vi "Ctor.vi"(8 "error in (no error)":errorcluster) -> (0 "error out":errorcluster, 3 "PlatformManager out":refnum<class "PlatformManager.lvclass">)   [LabVIEW 2020, in "PicoG-Core.lvlib" / "PlatformManager.lvclass"]
uses:
  PlatformManager.lvclass
  Ref Data.ctl
  Platform/Platform.lvclass
  PlatformManager.lvclass/PlatformManager.ctl
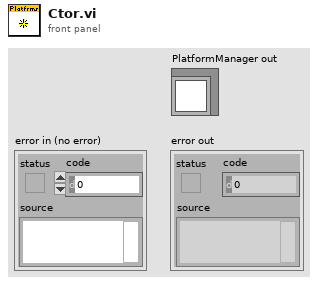
[diagram p1: front panel]
types:
  T1 = typedef "PicoG-Core.lvlib/PlatformManager.lvclass/Ref Data.ctl" = cluster{"Platforms":refnum<class "Platform.lvclass">[]}
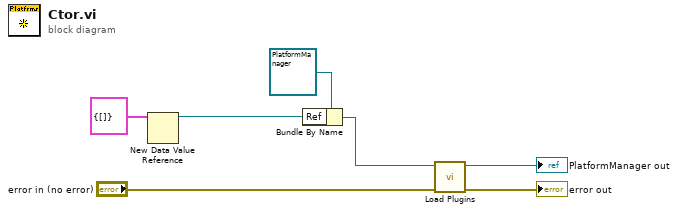
[diagram p0: block diagram]
diagram:
  n1 = New Data Value Reference(data value=T1 {"Platforms"=[]} ("Ref Data")) -> (data value reference=w5:refnum<data-value>)  [unwired: 1 in, 1 out]
  n2 = Bundle By Name(cluster=refnum<class "PlatformManager.lvclass"> refnum ("TargetPluginManager in"), "Ref"=w5) -> (w2:refnum<class "PlatformManager.lvclass">)
  n3 = call "Load Plugins.vi"("error in (no error)"="error in (no error)", "PlatformManager in"=w2) -> ("error out"=→"error out":errorcluster, "PlatformManager out"=→"PlatformManager out":refnum<class "PlatformManager.lvclass">)  [unwired: 8 in]
